vi "XYZ_sequence_generator_with_flags.vi"(8 "X-direction":enum16{"Up", "Down"}(ring), 9 "Y-direction":enum16{"Left", "Right"}(ring)=enum."Right", 11 "Acquisition":T1={"Acquire"=FALSE, "Step size X and Y (um)"=503.04, "Number of tiles in X"=1.0, "Number of tiles in Y"=1.0, "Number of slices in Z"=1.0, "Step size Z (um)"=0.2, "Image acquisition time (ms)"=1000.0, "Flyback time (ms)"=25.0, "Moving time between tiles (ms)"=5000.0, "Total progress"=0, "Percentage overlap"=5.0, "Voice coil calibration file"=path "", "Saved file location"=path "", "typedef_laser_order_control"={"Laser 560 nm order selection"=0, "Laser 595 nm order selection"=0, "Laser 642 nm order selection"=0, "Laser 488 nm order selection"=1, "Color Box"=60927, "Color Box 2"=12844800, "Color Box 3"=14132992, "Color Box 4"=16715008}, "Z-stack progress"=0} {"Z-stack progress" scale=0.0..100.0; "typedef_laser_order_control"."Laser 488 nm order selection" items=["Not active", "1", "2", "3", "4"]; "typedef_laser_order_control"."Laser 642 nm order selection" items=["Not active", "1", "2", "3", "4"]; "typedef_laser_order_control"."Laser 595 nm order selection" items=["Not active", "1", "2", "3", "4"]; "typedef_laser_order_control"."Laser 560 nm order selection" items=["Not active", "1", "2", "3", "4"]; "Percentage overlap" min=0.1 max=100.0; "Total progress" scale=0.0..100.0}) -> (2 "Laser order":string[](array[string]), 3 "string array":string[](array[string]))   [LabVIEW 2020]
uses:
  typedefs/typedef_acquisition.ctl
  typedefs/typedef_laser_order_control.ctl
panel:
  out "String 2":string
  out "appended array":u16[](array[numeric])
  out "Total number of tiles":dbl
  out "String":string
  in  "fast axis":enum16{"", "X-axis", "Y-axis"}(ring)
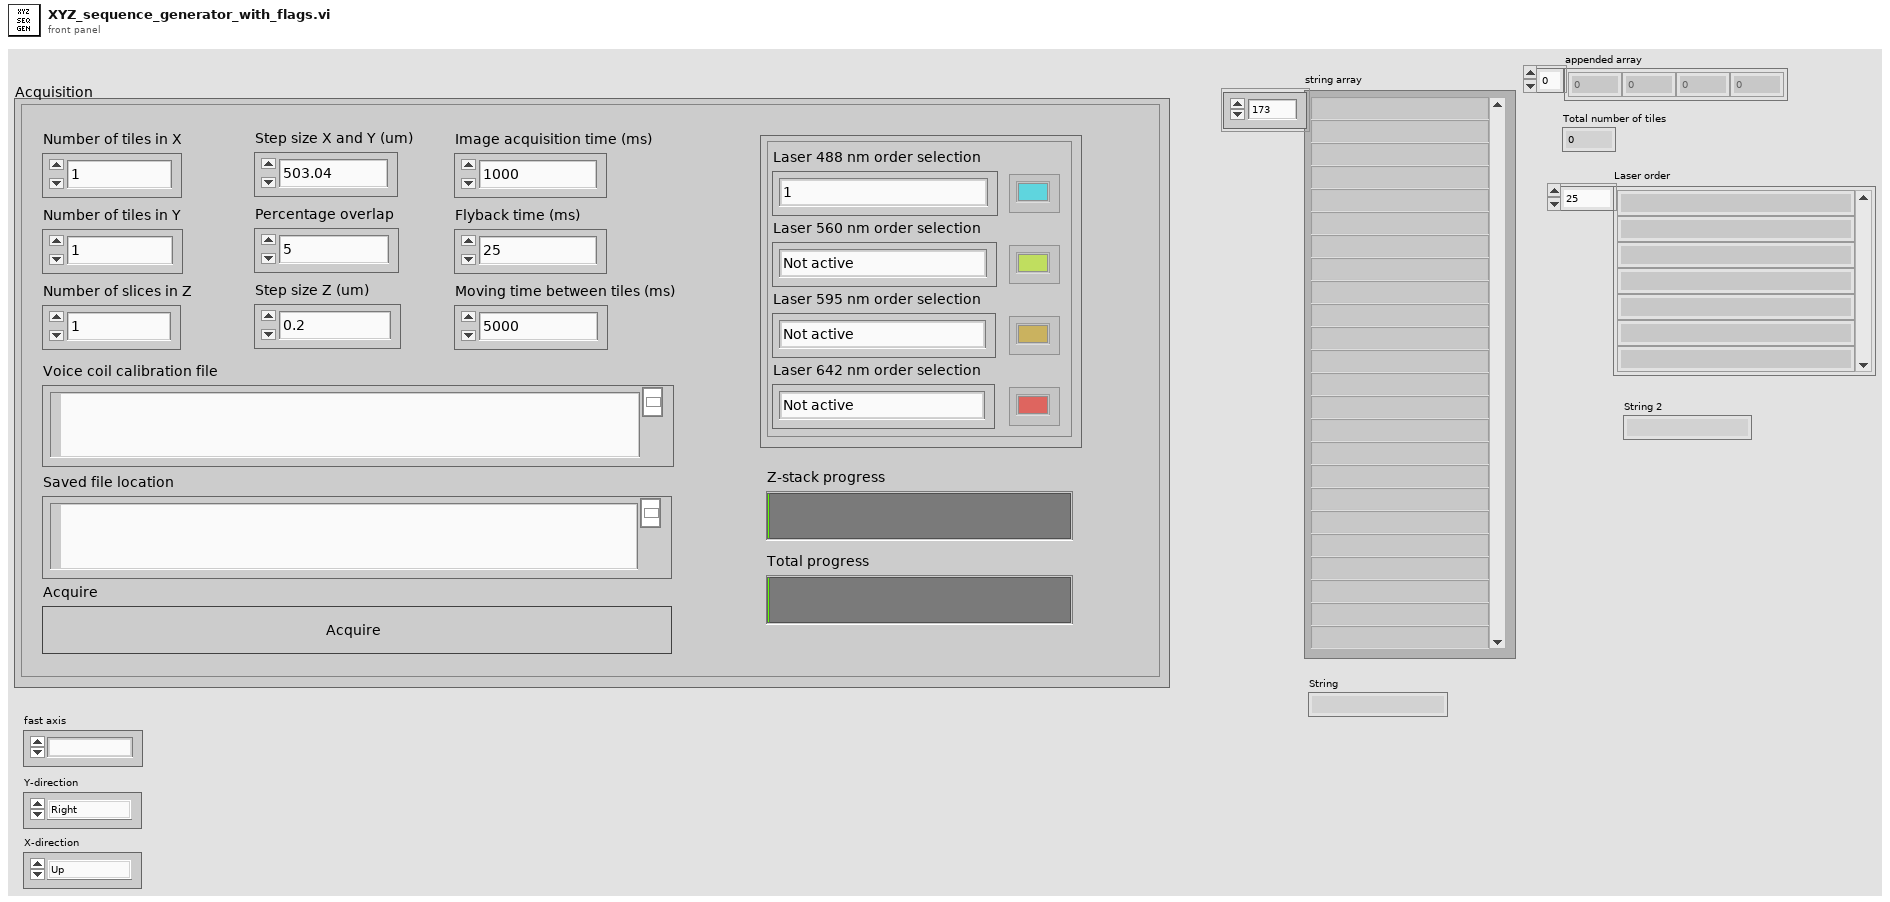
[diagram p1: front panel]
types:
  T1 = typedef "typedef_acquisition.ctl" = cluster{"Acquire":bool, "Step size X and Y (um)":dbl, "Number of tiles in X":dbl, "Number of tiles in Y":dbl, "Number of slices in Z":dbl, "Step size Z (um)":dbl, "Image acquisition time (ms)":dbl, "Flyback time (ms)":dbl, "Moving time between tiles (ms)":dbl, "Total progress":u8, "Percentage overlap":dbl, "Voice coil calibration file":path, "Saved file location":path, "typedef_laser_order_control":T2, "Z-stack progress":u8}
  T2 = typedef "typedef_laser_order_control.ctl" = cluster{"Laser 560 nm order selection":u16, "Laser 595 nm order selection":u16, "Laser 642 nm order selection":u16, "Laser 488 nm order selection":u16, "Color Box":u32, "Color Box 2":u32, "Color Box 3":u32, "Color Box 4":u32}
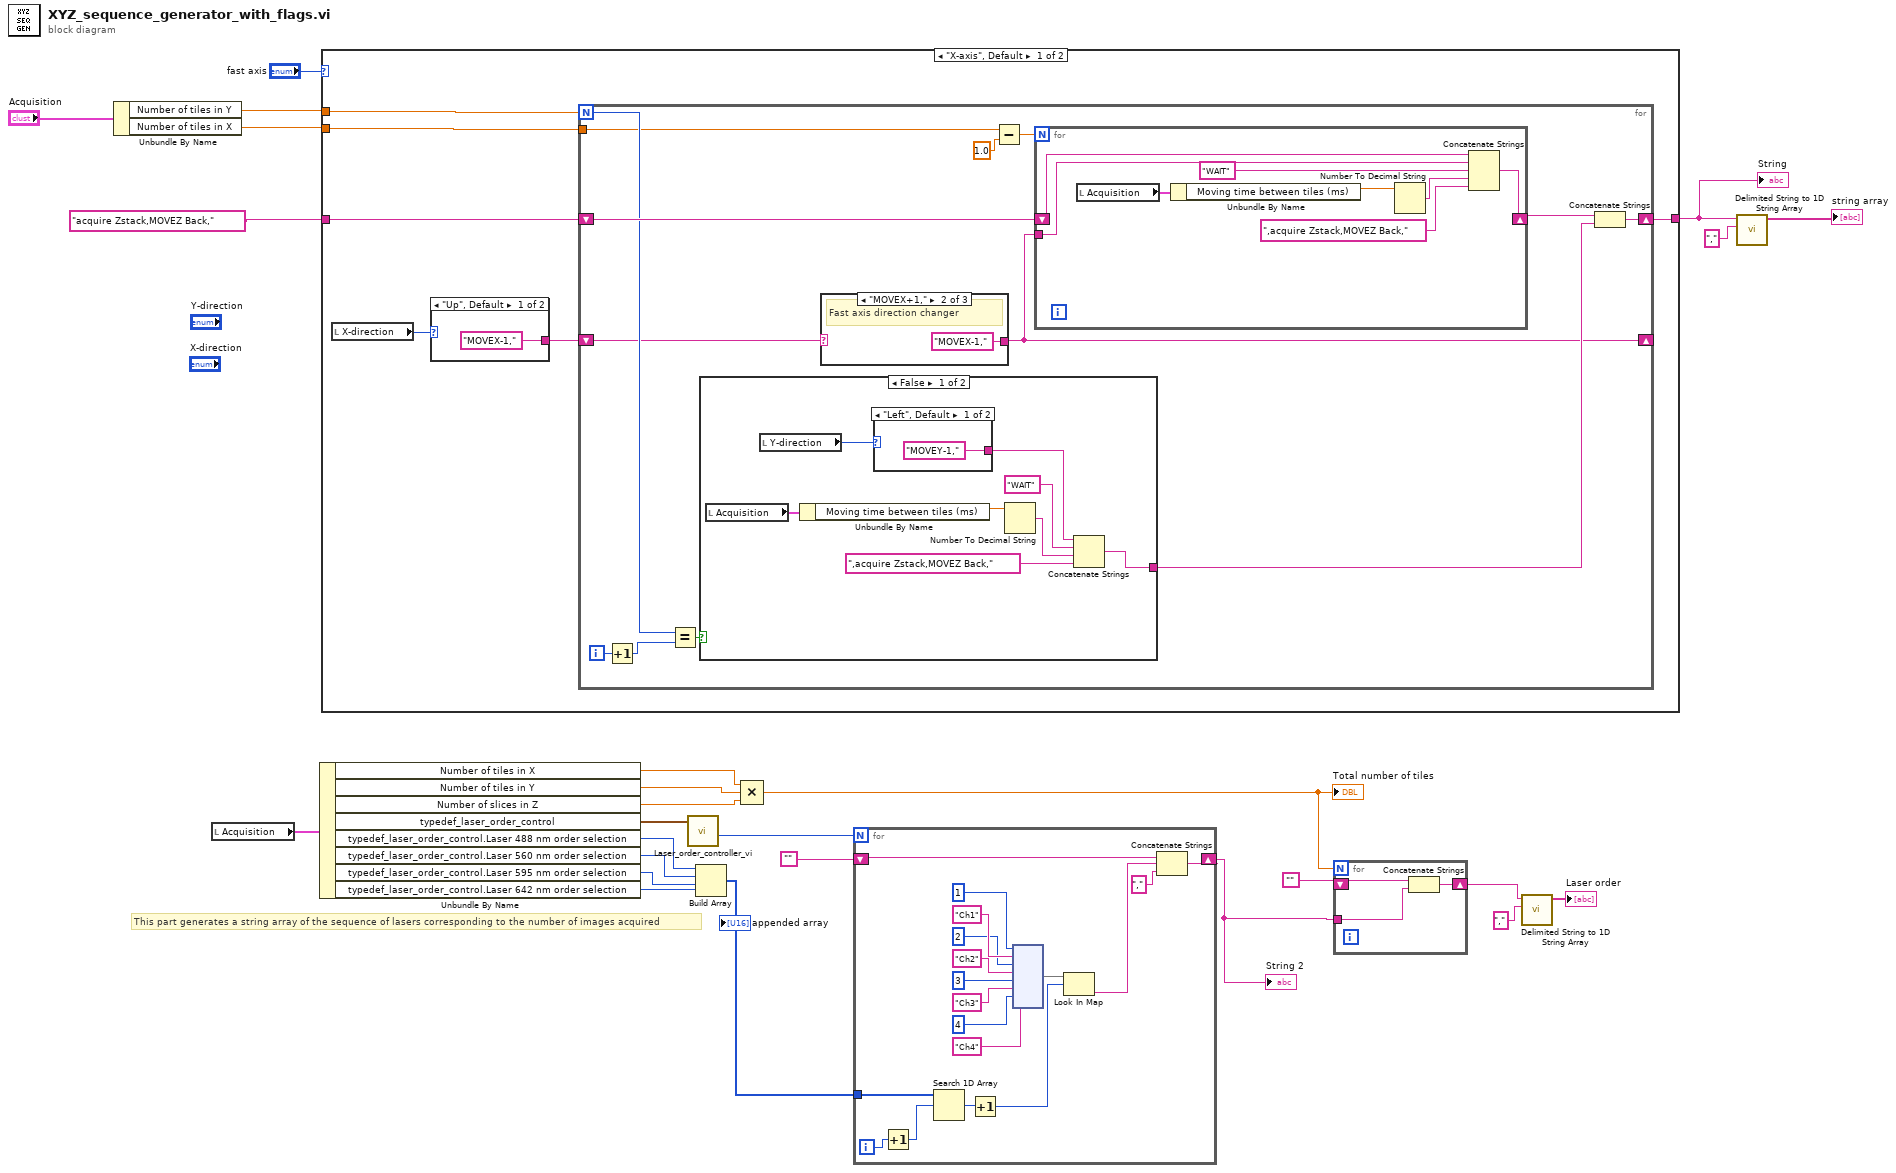
[diagram p0: block diagram]
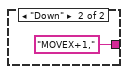
[diagram p2: hidden frame]
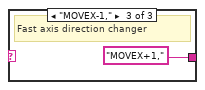
[diagram p4: hidden frame]
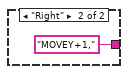
[diagram p5: hidden frame]
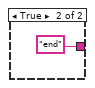
[diagram p6: hidden frame]
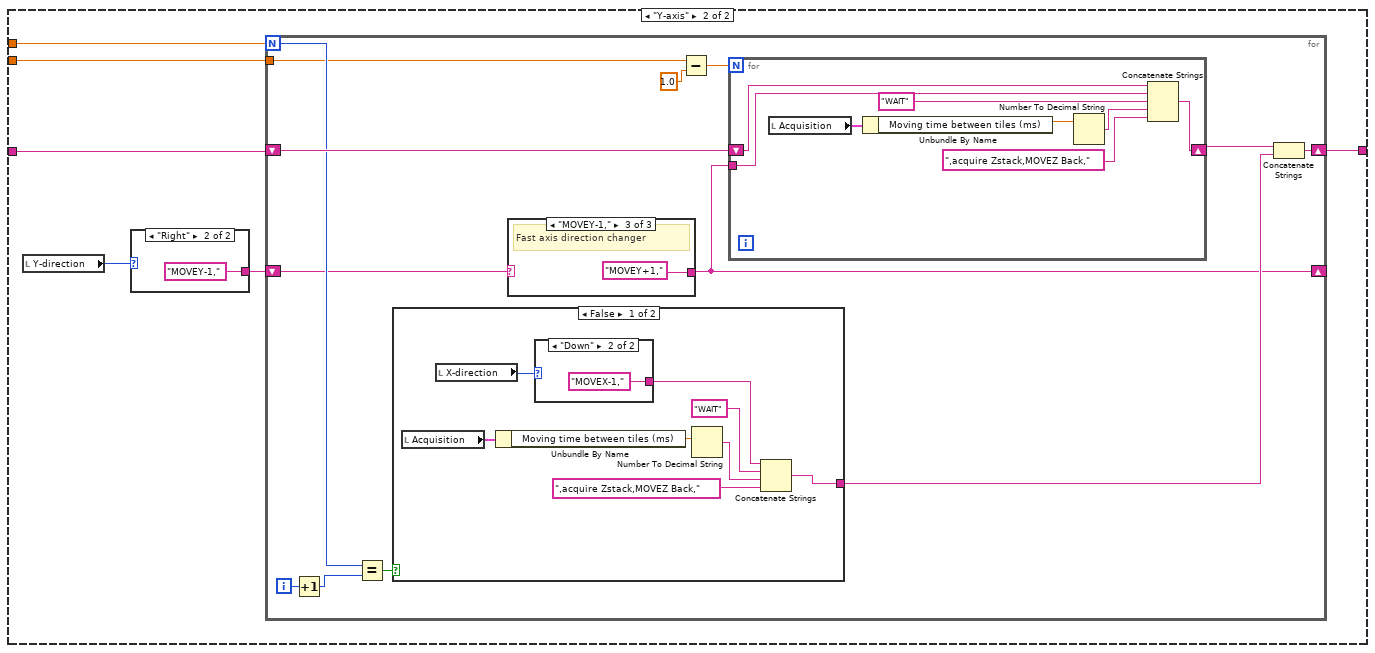
[diagram p7: hidden frame]
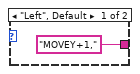
[diagram p8: hidden frame]
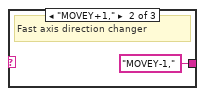
[diagram p10: hidden frame]
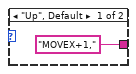
[diagram p11: hidden frame]
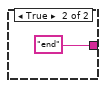
[diagram p12: hidden frame]
diagram:
  # "This part generates a string array of the sequence of lasers corresponding to the number of images acquired"
  n1 = Unbundle By Name("Acquisition") -> ("Number of tiles in Y"=w22:dbl, "Number of tiles in X"=w23:dbl)
  n2 = local read "Acquisition"() -> (w18:T1)
  n3 = Unbundle By Name(w18) -> ("Number of tiles in X"=w17:dbl, "Number of tiles in Y"=w16:dbl, "Number of slices in Z"=w15:dbl, "typedef_laser_order_control"=w14:T2, "typedef_laser_order_control.Laser 488 nm order selection"=w13:u16, "typedef_laser_order_control.Laser 560 nm order selection"=w12:u16, "typedef_laser_order_control.Laser 595 nm order selection"=w11:u16, "typedef_laser_order_control.Laser 642 nm order selection"=w10:u16)
  n4 = case shown="\"X-axis\", Default" "fast axis" {
    tunnel: [w32 w74] -> w26
    tunnel: w23 -> [w31 w73]
    tunnel: w22 -> [w30 w72]
    tunnel: "acquire Zstack,MOVEZ Back," -> [w29 w71]
    frame "X-axis", Default {
      n5 = local read "X-direction"() -> (w28:enum16{"Up", "Down"})
      n6 = case shown="\"Up\", Default" w28 {
        tunnel: ["MOVEX-1," "MOVEX+1,"] -> w27
        frame "Up", Default {
        }
        frame "Down" {
        }
      }
      n7 = for {
        N: w30 -> [w43]
        tunnel: w31 -> [w36]
        shift-right: [w45] -> w32
        shift-left: w29 -> [w47]
        shift-right: [w38] -> _
        shift-left: w27 -> [w39]
        i -> [w40]
        n8 = Increment(x=w40) -> (x+1=w41:i32)
        n9 = Equal?(x=w43, y=w41) -> (x = y?=w44:bool)
        n10 = case shown="False" w44 {
          tunnel: [w55 "end" ("string")] -> w42
          frame False {
            n11 = local read "Acquisition"() -> (w50:T1)
            n12 = local read "Y-direction"() -> (w53:enum16{"Left", "Right"})
            n13 = Unbundle By Name(w50) -> ("Moving time between tiles (ms)"=w57:dbl)
            n14 = case shown="\"Left\", Default" w53 {
              tunnel: ["MOVEY-1," "MOVEY+1,"] -> w52
              frame "Left", Default {
              }
              frame "Right" {
              }
            }
            n15 = Number To Decimal String(number=w57) -> (decimal integer string=w56:string)  [unwired: 1 in]
            n16 = Concatenate Strings(w52, "WAIT" ("string"), w56, ",acquire Zstack,MOVEZ Back,") -> (w55:string)
          }
          frame True {
          }
        }
        n17 = case shown="\"MOVEX+1,\"" w39 {
          tunnel: [_ "MOVEX-1," "MOVEX+1,"] -> w38
          frame "False", Default {
          }
          frame "MOVEX+1," {
            # "Fast axis direction changer"
          }
          frame "MOVEX-1," {
            # "Fast axis direction changer"
          }
        }
        n18 = Subtract(x=w36, y=1.0) -> (x-y=w37:dbl)
        n19 = for {
          N: w37 -> [_]
          shift-right: [w68] -> w46
          shift-left: w47 -> [w67]
          tunnel: w38 -> [w66]
          n20 = local read "Acquisition"() -> (w62:T1)
          n21 = Unbundle By Name(w62) -> ("Moving time between tiles (ms)"=w61:dbl)
          n22 = Number To Decimal String(number=w61) -> (decimal integer string=w64:string)  [unwired: 1 in]
          n23 = Concatenate Strings(w67, w66, "WAIT" ("string"), w64, ",acquire Zstack,MOVEZ Back,") -> (w68:string)
        }
        n24 = Concatenate Strings(w46, w42) -> (w45:string)
      }
    }
    frame "Y-axis" {
      n25 = local read "Y-direction"() -> (w70:enum16{"Left", "Right"})
      n26 = case shown="\"Right\"" w70 {
        tunnel: ["MOVEY+1," "MOVEY-1,"] -> w69
        frame "Left", Default {
        }
        frame "Right" {
        }
      }
      n27 = for {
        N: w72 -> [w85]
        tunnel: w73 -> [w78]
        shift-right: [w87] -> w74
        shift-left: w71 -> [w89]
        shift-right: [w80] -> _
        shift-left: w69 -> [w81]
        i -> [w82]
        n28 = Increment(x=w82) -> (x+1=w83:i32)
        n29 = Equal?(x=w85, y=w83) -> (x = y?=w86:bool)
        n30 = case shown="False" w86 {
          tunnel: [w98 "end" ("string")] -> w84
          frame False {
            n31 = local read "Acquisition"() -> (w93:T1)
            n32 = local read "X-direction"() -> (w96:enum16{"Up", "Down"})
            n33 = Unbundle By Name(w93) -> ("Moving time between tiles (ms)"=w92:dbl)
            n34 = case shown="\"Down\"" w96 {
              tunnel: ["MOVEX+1," "MOVEX-1,"] -> w95
              frame "Up", Default {
              }
              frame "Down" {
              }
            }
            n35 = Number To Decimal String(number=w92) -> (decimal integer string=w99:string)  [unwired: 1 in]
            n36 = Concatenate Strings(w95, "WAIT" ("string"), w99, ",acquire Zstack,MOVEZ Back,") -> (w98:string)
          }
          frame True {
          }
        }
        n37 = case shown="\"MOVEY-1,\"" w81 {
          tunnel: [_ "MOVEY-1," "MOVEY+1,"] -> w80
          frame "False", Default {
          }
          frame "MOVEY+1," {
            # "Fast axis direction changer"
          }
          frame "MOVEY-1," {
            # "Fast axis direction changer"
          }
        }
        n38 = Subtract(x=w78, y=1.0) -> (x-y=w79:dbl)
        n39 = for {
          N: w79 -> [_]
          shift-right: [w110] -> w88
          shift-left: w89 -> [w109]
          tunnel: w80 -> [w108]
          n40 = local read "Acquisition"() -> (w104:T1)
          n41 = Unbundle By Name(w104) -> ("Moving time between tiles (ms)"=w103:dbl)
          n42 = Number To Decimal String(number=w103) -> (decimal integer string=w106:string)  [unwired: 1 in]
          n43 = Concatenate Strings(w109, w108, "WAIT" ("string"), w106, ",acquire Zstack,MOVEZ Back,") -> (w110:string)
        }
        n44 = Concatenate Strings(w88, w84) -> (w87:string)
      }
    }
  }
  "String" <- w26
  n45 = call "Laser_order_controller_vi.vi"("typedef_laser_order_control"=w14) -> ("Active lasers"=w7:i16)  [unwired: 8 in, 2 out]
  n46 = Build Array(w13, w12, w11, w10) -> (w8:u16[])
  "appended array" <- w8
  n47 = Compound Arithmetic op=MULTIPLY(w17, w16, w15) -> (w6:dbl)
  "Total number of tiles" <- w6
  n48 = for {
    N: w7 -> [_]
    tunnel: w8 -> [w114]
    shift-right: [w117] -> w5
    shift-left: "" -> [w119]
    i -> [w116]
    n49 = Increment(x=w116) -> (x+1=w115:i32)
    n50 = Search 1D Array(1D array=w114, element=w115) -> (index of element=w113:i32)  [unwired: 1 in]
    n51 = Increment(x=w113) -> (x+1=w112:i32)
    n52 = node(1 ("value"), "Ch1" ("key"), 2 ("value"), "Ch2" ("key"), 3 ("value"), "Ch3" ("key"), 4 ("value"), "Ch4" ("key")) -> (w128:map{i32, string})
    n53 = Look In Map(map=w128, key=w112) -> (value=w118:string)  [unwired: 1 in, 1 out]
    n54 = Concatenate Strings(w119, w118, "," ("string")) -> (w117:string)
  }
  "String 2" <- w5
  n55 = for {
    N: w6 -> [_]
    shift-right: [w129] -> w4
    shift-left: "" -> [w131]
    tunnel: w5 -> [w130]
    n56 = Concatenate Strings(w131, w130) -> (w129:string)
  }
  n57 = call <vilib>:"Delimited String to 1D String Array.vi"("delimiter"=",", "delimited string"=w4) -> ("string array"=→"Laser order":string[])  [unwired: 9 in]
  n58 = call <vilib>:"Delimited String to 1D String Array.vi"("delimiter"=",", "delimited string"=w26) -> ("string array"=→"string array":string[])  [unwired: 9 in]
